vi "Write Target Name.vi"(8 "error in (no error)":errorcluster, 10 "Target Name":string, 11 "Set Version from Git Tag in":refnum<class "Set Version from Git Tag.lvclass">) -> (0 "error out":errorcluster, 3 "Set Version from Git Tag out":refnum<class "Set Version from Git Tag.lvclass">)   [LabVIEW 2020, in "ProjectBuilder.lvlib" / "Set Version from Git Tag.lvclass"]
doc: "Write 'Target Name' to the private data."
uses:
  Set Version from Git Tag.lvclass
  Set Version from Git Tag.lvclass/Set Version from Git Tag.ctl
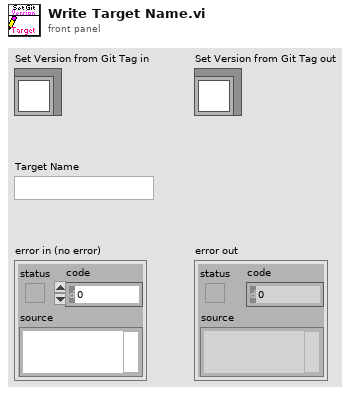
[diagram p1: front panel]
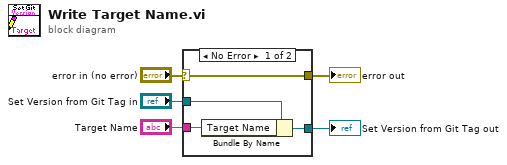
[diagram p0: block diagram]
diagram:
  n1 = case shown="No Error" "error in (no error)" {
    selector: "error in (no error)" -> [w9 w10]
    tunnel: [w9 w10] -> w4
    tunnel: [w7 w11] -> w2
    tunnel: "Set Version from Git Tag in" -> [w8 w11]
    tunnel: "Target Name" -> [w6 _]
    frame No Error {
      n2 = Bundle By Name(cluster=w8, "Target Name"=w6) -> (w7:refnum<class "Set Version from Git Tag.lvclass">)
    }
    frame Error {
    }
  }
  "error out" <- w4
  "Set Version from Git Tag out" <- w2
